vi "Process Tree Hover.vi"(9 "Coords":T1, 10 "Search Results":T4(array[cluster]), 11 "TreeControl in":refnum<vi>) -> ()   [LabVIEW 2019]
uses:
  Advanced Search.llb/Terminal Filter Output.ctl
  Advanced Search.llb/Terminals within Selection and GObject.ctl
  <vilib>/Utility/miscctls.llb/LVPoint32TypeDef.ctl
  <vilib>/Utility/inputDevices.llb/mouseAcquire.vi
  <vilib>/Utility/inputDevices.llb/closeMouse.vi
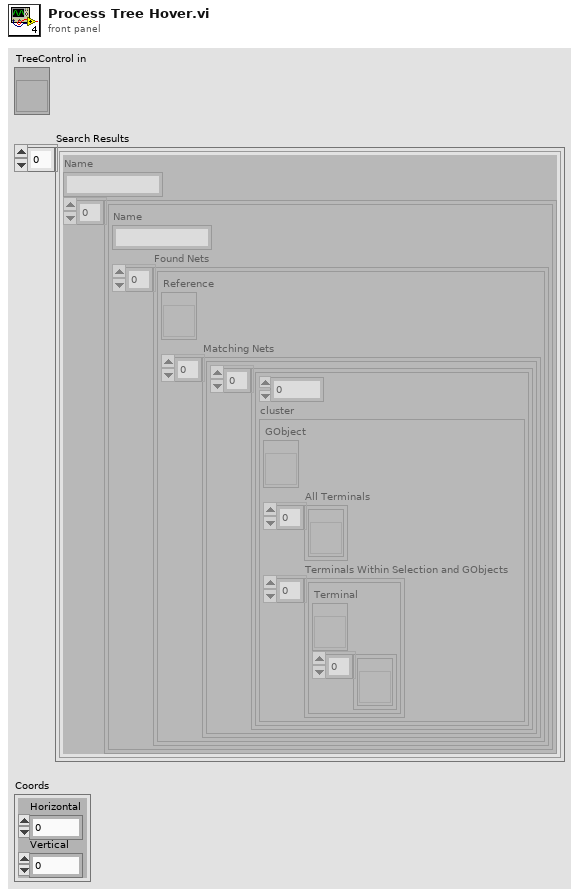
[diagram p1: front panel]
types:
  T1 = typedef "LVPoint32TypeDef.ctl" = cluster{"Horizontal":i32, "Vertical":i32}
  T2 = typedef "Terminal Filter Output.ctl" = cluster{"GObject":refnum<vi>, "All Terminals":refnum<vi>[], "Terminals Within Selection and GObjects":T3[]}
  T3 = typedef "Terminals within Selection and GObject.ctl" = cluster{"Terminal":refnum<vi>, "Attached GObjects":refnum<vi>[]}
  T4 = cluster{"Name":string, cluster{"Name":string, "Found Nets":cluster{"Reference":refnum<vi>, "Matching Nets":cluster{cluster{i32, "cluster":T2}[]}[]}[]}[]}[]
  T5 = cluster{"Name":string, "Found Nets":cluster{"Reference":refnum<vi>, "Matching Nets":cluster{cluster{i32, "cluster":T2}[]}[]}[]}[]
  T6 = cluster{"Reference":refnum<vi>, "Matching Nets":cluster{cluster{i32, "cluster":T2}[]}[]}[]
  T7 = cluster{"Horizontal":i32, "Vertical":i32, "Scrolling":i32}
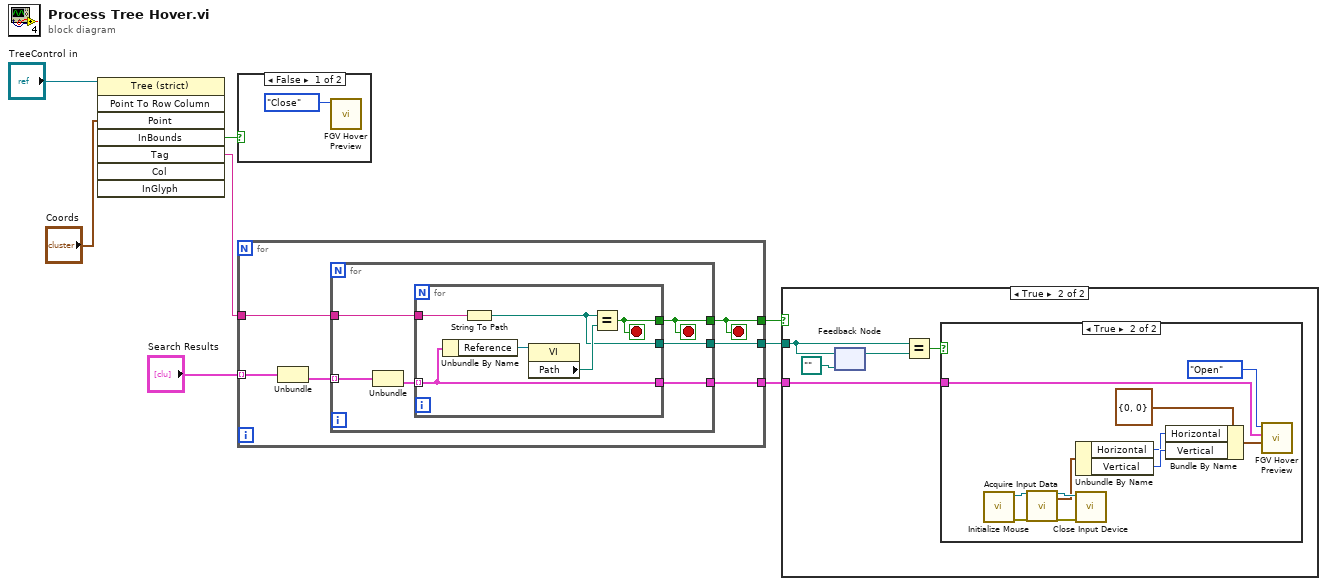
[diagram p0: block diagram]
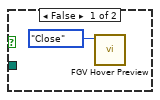
[diagram p3: hidden frame]
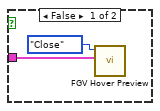
[diagram p4: hidden frame]
diagram:
  n1 = invoke class="Tree (strict)" method="Point To Row Column"(reference="TreeControl in", "Point"="Coords") -> ("InBounds"=w7:bool, "Tag"=w2:string)  [unwired: 6 in, 6 out]
  n2 = case shown="False" w7 {
    frame False {
      n3 = call "FGV Hover Preview.vi"("Command"=enum16{"Open", "Close", "Tick"}."Close") -> ()  [unwired: 11 in]
    }
    frame True {
    }
  }
  n4 = for {
    tunnel: "Search Results" -> [w15] mode=indexing
    tunnel: w2 -> [w13]
    tunnel: [w10] -> w3
    tunnel: [w12] -> w4
    tunnel: [w11] -> w5
    stop <- w10 stop-if-true
    n5 = Unbundle(w15) -> (w14:T5)  [unwired: 1 out]
    n6 = for {
      tunnel: w14 -> [w21] mode=indexing
      tunnel: w13 -> [w19]
      tunnel: [w16] -> w10
      tunnel: [w18] -> w12
      tunnel: [w17] -> w11
      stop <- w16 stop-if-true
      n7 = Unbundle(w21) -> ("Found Nets"=w20:T6)  [unwired: 1 out]
      n8 = for {
        tunnel: w20 -> [w24] mode=indexing
        tunnel: w19 -> [w25]
        tunnel: [w22] -> w16
        tunnel: [w24] -> w18
        tunnel: [w23] -> w17
        stop <- w22 stop-if-true
        n9 = Unbundle By Name(w24) -> ("Reference"=w27:refnum<vi>)
        n10 = String To Path(string=w25) -> (path=w23:path)
        n11 = property class="VI"(reference=w27) -> ("Path"=w26:path)  [unwired: 1 in, 2 out]
        n12 = Equal?(x=w23, y=w26) -> (x = y?=w22:bool)
      }
    }
  }
  n13 = case shown="True" w3 {
    tunnel: w4 -> [_ w33]
    tunnel: w5 -> [_ w32]
    frame False {
      n14 = call "FGV Hover Preview.vi"("Command"=enum16{"Open", "Close", "Tick"}."Close") -> ()  [unwired: 11 in]
    }
    frame True {
      n15 = feedback #1(path "") -> (w29:path)
      n16 = feedback-in #1(w32) -> ()
      n17 = Equal?(x=w32, y=w29) -> (x = y?=w31:bool)
      n18 = case shown="True" w31 {
        tunnel: w33 -> [w34 w46]
        frame False {
          n19 = call "FGV Hover Preview.vi"("Net Data"=w34, "Command"=enum16{"Open", "Close", "Tick"}."Close") -> ()  [unwired: 10 in]
        }
        frame True {
          n20 = call <vilib>:"Initialize Mouse.vi"() -> ("error out"=w43:errorcluster, "device ID"=w44:refnum<k1>)  [unwired: 10 in]
          n21 = call-poly <vilib>:"Acquire Input Data.vi"("device ID"=w44, "error in (no error)"=w43) -> ("device ID"=w42:refnum<k1>, "axis info"=w40:T7, "error out"=w41:errorcluster)  [unwired: 14 in, 1 out]
          n22 = Unbundle By Name(w40) -> ("Horizontal"=w36:i32, "Vertical"=w37:i32)
          n23 = call-poly <vilib>:"Close Input Device.vi"("error in (no error)"=w41, "device ID"=w42) -> ()  [unwired: 8 in, 1 out]
          n24 = Bundle By Name(cluster=T1 {"Horizontal"=0, "Vertical"=0} ("Mouse Coordinates"), "Horizontal"=w36, "Vertical"=w37) -> (w38:T1)
          n25 = call "FGV Hover Preview.vi"("Mouse Coordinates"=w38, "Net Data"=w46, "Command"=enum16{"Open", "Close", "Tick"}."Open") -> ()  [unwired: 9 in]
        }
      }
    }
  }
